vi "Write Temperature Test Results.vi"(8 "Actual Temperature":dbl, 9 "Pass Fail":bool, 10 "MTS Temperature":dbl) -> ()   [LabVIEW 2015, in "LCM Single-Up MTS Test.lvclass"]
uses:
  LCM Single-Up MTS Test.lvclass
  <vilib>/Cree, Inc/Cree Test Framework/Core Launcher/Core Manager Methods -- Enum.ctl
  <vilib>/Cree, Inc/Cree Test Framework/Classes/Data/Data Repo/Class/Data Repo.lvclass
  <vilib>/Cree, Inc/Cree Test Framework/Core Launcher/Core Launcher.lvlib
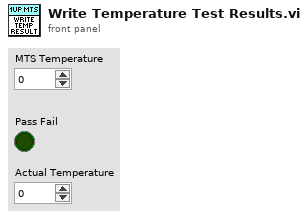
[diagram p1: front panel]
types:
  T1 = typedef "Core Launcher.lvlib/Core Manager Methods -- Enum.ctl" = enum16{"Spawn Objects", "Get Objects", "Destroy Objects"}
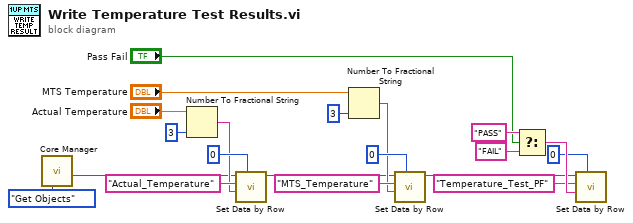
[diagram p0: block diagram]
diagram:
  n1 = call <vilib>:"Core Manager.vi"("Method"=Core_Manager_Methods_--_Enum."Get Objects") -> ("Data Repo"=w3:refnum<class "Data Repo.lvclass">)  [unwired: 7 in, 3 out]
  n2 = Number To Fractional String(number="Actual Temperature", precision (6)=i16 3) -> (F-format string=w6:string)  [unwired: 2 in]
  n3 = call <vilib>:"Set Data by Row.vi"("Row"=0, "Value"=w6, "Header"="Actual_Temperature", "Acrobat Template in"=w3) -> ("Acrobat Template out"=w2:refnum<class "Data Repo.lvclass">)  [unwired: 6 in, 1 out]
  n4 = Number To Fractional String(number="MTS Temperature", precision (6)=i16 3) -> (F-format string=w10:string)  [unwired: 2 in]
  n5 = call <vilib>:"Set Data by Row.vi"("Row"=0, "Value"=w10, "Header"="MTS_Temperature", "Acrobat Template in"=w2) -> ("Acrobat Template out"=w1:refnum<class "Data Repo.lvclass">)  [unwired: 6 in, 1 out]
  n6 = Select(t="PASS" ("Header"), s="Pass Fail", f="FAIL" ("Header")) -> (s? t:f=w20:string)
  n7 = call <vilib>:"Set Data by Row.vi"("Row"=0, "Value"=w20, "Header"="Temperature_Test_PF", "Acrobat Template in"=w1) -> ()  [unwired: 6 in, 2 out]
